vi "Read I64.vi"(7 "Channel Index":i32, 8 "error in (no error)":errorcluster, 11 "CIFCorePlugin in":refnum<class "CIFCorePlugin.lvclass">) -> (0 "error out":errorcluster, 2 "Data":i64, 3 "CIFCorePlugin out":refnum<class "CIFCorePlugin.lvclass">)   [LabVIEW 2021, in "CIFCorePlugin.lvclass"]
uses:
  CIFCorePlugin.lvclass
  CIFCorePlugin.lvclass/CIFCorePlugin.ctl
  CIFUtilities/CIFChannelMng/CIFChannelMng.lvclass/CIFChannelMng.ctl
  CIFUtilities/CIFChannelMng/Accessors/Read Channel Array.vi
  CIFUtilities/CIFChannelMng/Accessors/Write Channel Array.vi
  CIFUtilities/CIFChannels/CIFChannels.lvclass
  CIFUtilities/CIFChannelMng/CIFChannelMng.lvclass
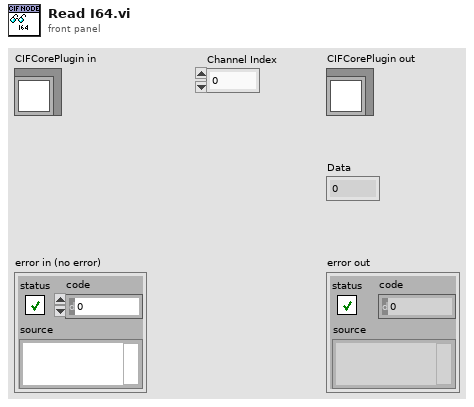
[diagram p1: front panel]
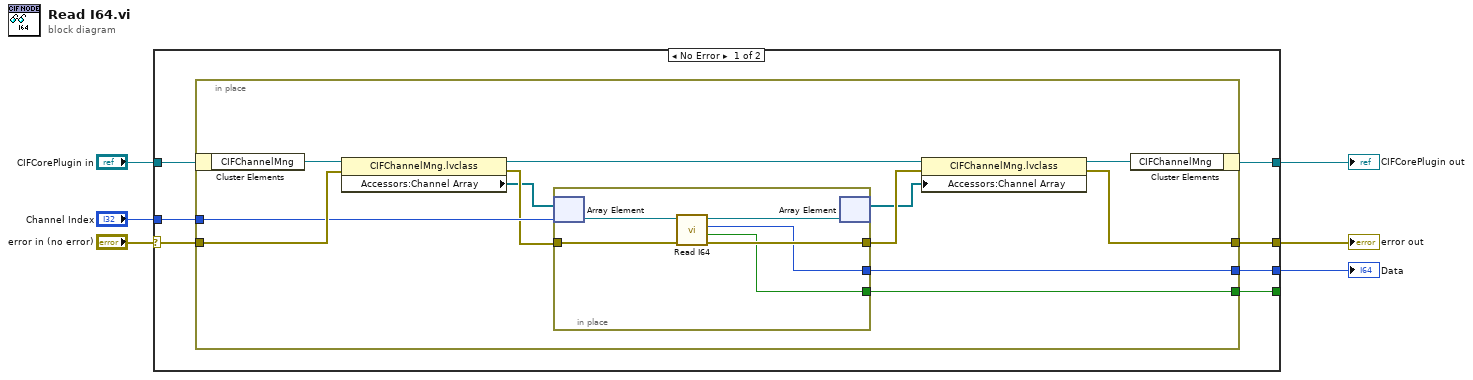
[diagram p0: block diagram]
diagram:
  n1 = case shown="No Error" "error in (no error)" {
    selector: "error in (no error)" -> [w13 w33]
    tunnel: [w12 w33] -> w3
    tunnel: [w8 w32] -> w4
    tunnel: "CIFCorePlugin in" -> [w9 w32]
    tunnel: [w11 _] -> w2
    tunnel: [w10 _] -> _
    tunnel: "Channel Index" -> [w7 _]
    frame No Error {
      n2 = in-place {
        in-place-border: w13 -> [w21]
        in-place-border: [w14] -> w12
        in-place-border: [w25] -> w11
        in-place-border: [w24] -> w10
        in-place-border: w7 -> [w20]
        n3 = in-place-cluster #1(w9) -> ("CIFChannelMng"=w23:refnum<class "CIFChannelMng.lvclass">)
        n4 = property class="CIFChannelMng.lvclass"(reference=w23, error in=w21) -> (reference out=w19:refnum<class "CIFChannelMng.lvclass">, error out=w18:errorcluster, "Accessors:Channel Array"=w16:refnum<class "CIFChannels.lvclass">[])
        n5 = in-place {
          in-place-border: w18 -> [w30]
          in-place-border: [w29] -> w17
          in-place-border: [w28] -> w24
          in-place-border: [w27] -> w25
          n6 = in-place-array #2(w16, w20) -> (w31:refnum<class "CIFChannels.lvclass">)
          n7 = call-dynamic "Read I64.vi"("error in (no error)"=w30, "CIFChannels in"=w31) -> ("error out"=w29:errorcluster, "timed out?"=w28:bool, "Data"=w27:i64, "CIFChannels out"=w26:refnum<class "CIFChannels.lvclass">)  [unwired: 6 in]
          n8 = in-place-array #2(w26) -> (w15:refnum<class "CIFChannels.lvclass">[])  [unwired: 1 out]
        }
        n9 = property class="CIFChannelMng.lvclass"(reference=w19, error in=w17, "Accessors:Channel Array"=w15) -> (reference out=w22:refnum<class "CIFChannelMng.lvclass">, error out=w14:errorcluster)
        n10 = in-place-cluster #1("CIFChannelMng"=w22) -> (w8:refnum<class "CIFCorePlugin.lvclass">)
      }
    }
    frame Error {
    }
  }
  "error out" <- w3
  "CIFCorePlugin out" <- w4
  "Data" <- w2
